vi "Update Temp Setpoint.vi"(8 "error in (no error)":errorcluster, 10 "Setpoint (C)":dbl, 11 "Abstract Chamber in":refnum<class "Abstract Chamber.lvclass">) -> (0 "error out":errorcluster, 3 "Abstract Chamber out":refnum<class "Abstract Chamber.lvclass">)   [LabVIEW 2020, in "Chamber Controller.lvlib" / "Abstract Chamber.lvclass"]
uses:
  Abstract Chamber.lvclass
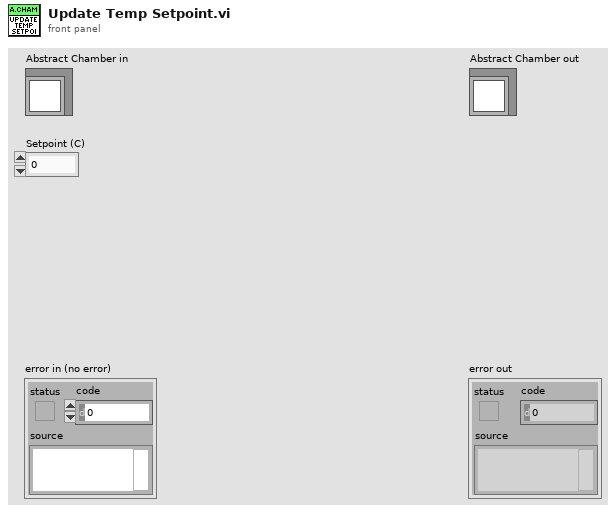
[diagram p1: front panel]
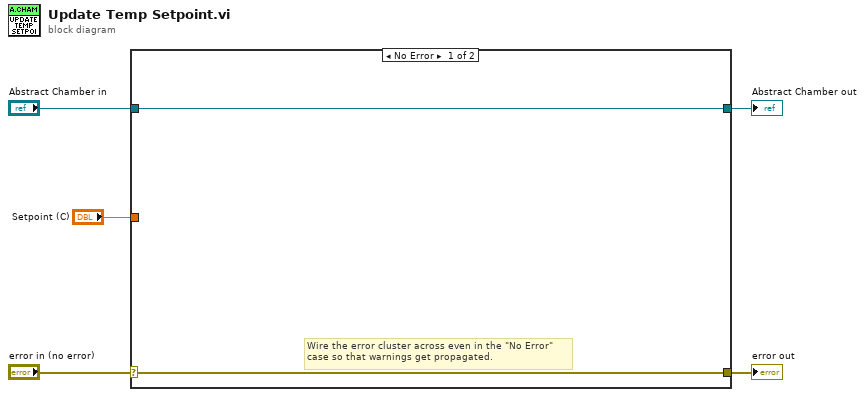
[diagram p0: block diagram]
diagram:
  n1 = case shown="No Error" "error in (no error)" {
    selector: "error in (no error)" -> [w6 w9]
    tunnel: [w6 w9] -> w4
    tunnel: [w7 w8] -> w2
    tunnel: "Abstract Chamber in" -> [w7 w8]
    tunnel: "Setpoint (C)" -> [_ _]
    frame No Error {
      # "Wire the error cluster across even in the \"No Error\"\ncase so that warnings get propagated."
    }
    frame Error {
    }
  }
  "error out" <- w4
  "Abstract Chamber out" <- w2
